vi "Set Value.vi"(0 "Diagram in":refnum<vi>, 1 "Sub Items":T1[](array[typedef]), 5 "Value in":refnum<vi>, 9 "Input Terms in":cluster{refnum<vi>, "Type":variant}[](array[cluster]), 11 "error in (no error)":errorcluster) -> (4 "Diagram out":refnum<vi>, 6 "Value out":refnum<vi>, 8 "Equal":refnum<vi>, 10 "Input Terms out":cluster{refnum<vi>, "Type":variant}[](array[cluster]), 15 "error out":errorcluster)   [LabVIEW 2015, in "Read-Write-Signals.xnode"]
uses:
  Read-Write-Signals.xnode
  Read-Write-Signals Sub Item.ctl
  Read-Write-Signals Sub Item Type.ctl
  <vilib>/Erdos Miller/LV-Scripting/LV-Scripting.lvlib
  <vilib>/Utility/Data Type/NI_Data Type.lvlib
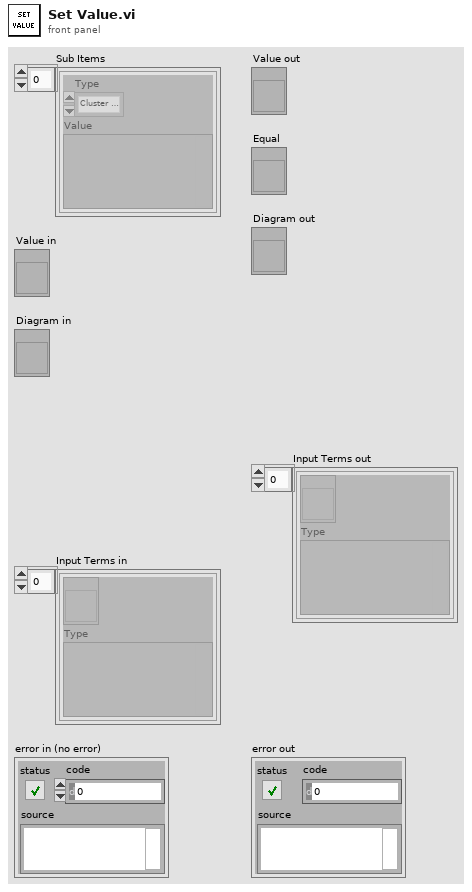
[diagram p1: front panel]
types:
  T1 = typedef "Read-Write-Signals Sub Item.ctl" = cluster{"Type":T2, "Value":variant}
  T2 = typedef "Read-Write-Signals Sub Item Type.ctl" = enum8{"Cluster Element", "Array Element", "Subarray"}
  T3 = cluster{"Outer Term":refnum<vi>, "Type":variant}[]
  T4 = typedef "NI_Data Type.lvlib/Data Type.ctl" = enum8{"Invalid Type", "Void", "I8", "I16", "I32", "I64", "U8", "U16", "U32", "U64", "Single Float", "Double Float", "Extended Float", "Single Complex", "Double Complex", "Extended Complex", "Enum U8", "Enum U16", "Enum U32", "Enum U64", "Single Float With Unit", "Double Float With Unit", "Extended Float With Unit", "Single Complex with Unit", "Double Complex with Unit", "Extended Complex with Unit", "Boolean", "String", "Path", "Picture", "Tag", "Array", "Cluster", "Variant", "LV Variant", "Waveform", "Timestamp", "Digital Waveform", "Digital Data", "ExpressData", "Refnum", "External Data", "VI", "Poly VI", "LabVIEW Class Instance", "Fixed Point"}
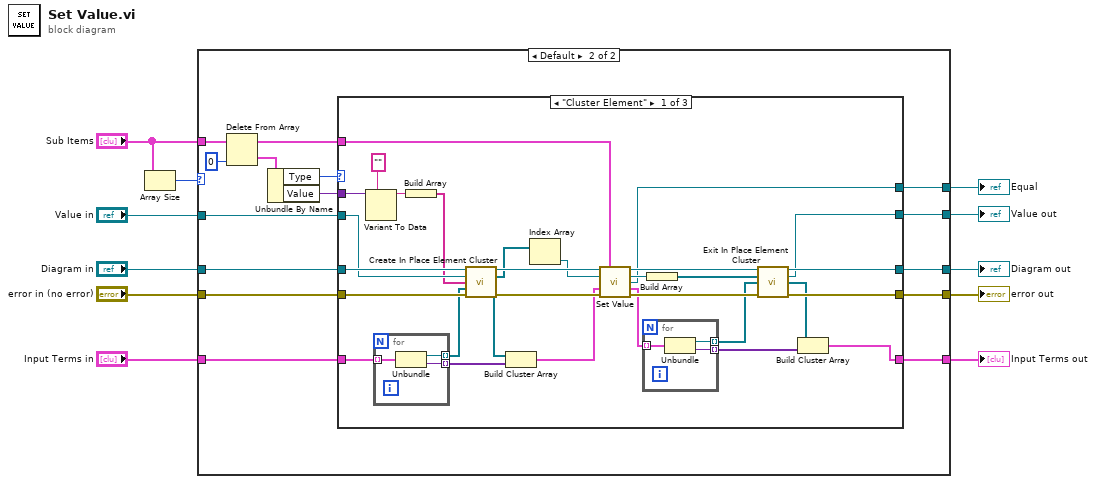
[diagram p0: block diagram]
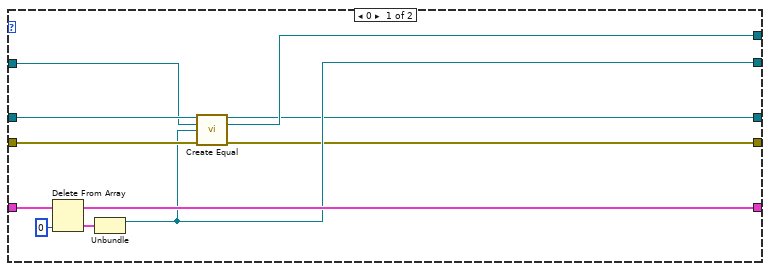
[diagram p2: hidden frame]
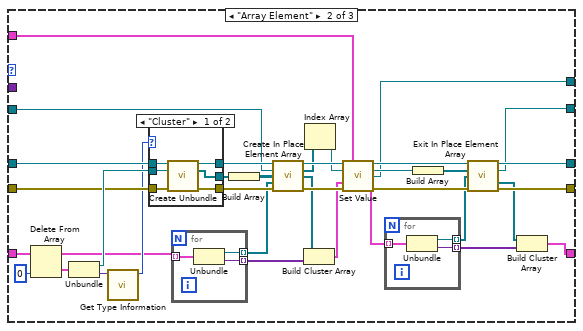
[diagram p3: hidden frame]
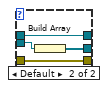
[diagram p4: hidden frame]
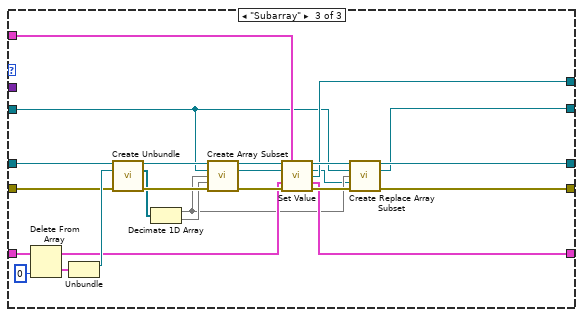
[diagram p5: hidden frame]
diagram:
  n1 = Array Size(array="Sub Items") -> (size(s)=w2:i32)
  n2 = case shown="Default" w2 {
    tunnel: [w14 w37] -> w11
    tunnel: "Sub Items" -> [_ w26]
    tunnel: [w15 w34] -> w10
    tunnel: [w12 w33] -> w9
    tunnel: "error in (no error)" -> [w22 w32]
    tunnel: "Diagram in" -> [w21 w31]
    tunnel: [w18 w30] -> w6
    tunnel: [w13 w29] -> w5
    tunnel: "Input Terms in" -> [w20 w28]
    tunnel: "Value in" -> [w16 w27]
    frame 0 {
      n3 = Delete From Array(array=w20, index=0) -> (deleted portion=w17:cluster{refnum<vi>, "Type":variant}, array with subset deleted=w18:cluster{refnum<vi>, "Type":variant}[])  [unwired: 1 in]
      n4 = Unbundle(w17) -> (w15:refnum<vi>)  [unwired: 1 out]
      n5 = call <vilib>:"Create Equal.vi"("Diagram in"=w21, "x"=w16, "y"=w15, "error in (no error)"=w22) -> ("Diagram out"=w12:refnum<vi>, "x = y?"=w14:refnum<vi>, "error out"=w13:errorcluster)  [unwired: 9 in]
    }
    frame Default {
      n6 = Delete From Array(array=w26, index=0) -> (deleted portion=w23:T1, array with subset deleted=w24:T1[])  [unwired: 1 in]
      n7 = Unbundle By Name(w23) -> ("Type"=w35:T2, "Value"=w36:variant)
      n8 = case shown="\"Cluster Element\"" w35 {
        tunnel: w36 -> [w67 _ _]
        tunnel: w28 -> [w47 w109 w150]
        tunnel: w31 -> [w64 w106 w147]
        tunnel: w32 -> [w63 w105 w146]
        tunnel: [w38 w74 w132] -> w30
        tunnel: [w52 w87 w140] -> w33
        tunnel: [w54 w85 w141] -> w29
        tunnel: w27 -> [w62 w98 w128]
        tunnel: [w48 w86 w129] -> w34
        tunnel: [w49 w84 w130] -> w37
        tunnel: w24 -> [w56 w95 w135]
        frame "Cluster Element" {
          n9 = Variant To Data(type="", Variant=w67) -> (data=w65:string)  [unwired: 1 in, 1 out]
          n10 = for {
            tunnel: w47 -> [w73] mode=indexing
            tunnel: [w72] -> w46 mode=indexing
            tunnel: [w71] -> w45 mode=indexing
            n11 = Unbundle(w73) -> (w72:refnum<vi>, "Type"=w71:variant)
          }
          n12 = Build Array(w65) -> (w61:string[])
          n13 = call <vilib>:"Create In Place Element Cluster.vi"("Diagram in"=w64, "Cluster"=w62, "Element Names"=w61, "Inputs"=w46, "error in (no error)"=w63) -> ("Diagram out"=w60:refnum<vi>, "Elements"=w59:refnum<vi>[], "Inputs"=w44:refnum<vi>[], "error out"=w57:errorcluster)  [unwired: 7 in]
          n14 = Build Cluster Array(w44, w45) -> (w43:cluster{refnum<vi>, "Type":variant}[])
          n15 = Index Array(array=w59) -> (element=w58:refnum<vi>)  [unwired: 1 in]
          n16 = call "Set Value.vi"("Diagram in"=w60, "Sub Items"=w56, "Value in"=w58, "Input Terms in"=w43, "error in (no error)"=w57) -> ("Diagram out"=w53:refnum<vi>, "Value out"=w51:refnum<vi>, "Equal"=w49:refnum<vi>, "Input Terms out"=w41:cluster{refnum<vi>, "Type":variant}[], "error out"=w55:errorcluster)  [unwired: 6 in]
          n17 = for {
            tunnel: w41 -> [w70] mode=indexing
            tunnel: [w69] -> w40 mode=indexing
            tunnel: [w68] -> w42 mode=indexing
            n18 = Unbundle(w70) -> (w69:refnum<vi>, "Type"=w68:variant)
          }
          n19 = Build Array(w51) -> (w50:refnum<vi>[])
          n20 = call <vilib>:"Exit In Place Element Cluster.vi"("Diagram in"=w53, "Elements"=w50, "Outputs"=w40, "error in (no error)"=w55) -> ("Diagram out"=w52:refnum<vi>, "Cluster"=w48:refnum<vi>, "Outputs"=w39:refnum<vi>[], "error out"=w54:errorcluster)  [unwired: 8 in]
          n21 = Build Cluster Array(w39, w42) -> (w38:T3)
        }
        frame "Array Element" {
          n22 = Delete From Array(array=w109, index=0) -> (deleted portion=w108:cluster{refnum<vi>, "Type":variant}, array with subset deleted=w82:cluster{refnum<vi>, "Type":variant}[])  [unwired: 1 in]
          n23 = Unbundle(w108) -> (w107:refnum<vi>, "Type"=w103:variant)
          n24 = call <vilib>:"Get Type Information.vi"("Variant"=w103) -> ("Type"=w102:T4)  [unwired: 6 in, 4 out]
          n25 = case shown="\"Cluster\"" w102 {
            tunnel: w107 -> [w119 w125]
            tunnel: w106 -> [w121 w123]
            tunnel: w105 -> [w120 w124]
            tunnel: [w117 w124] -> w100
            tunnel: [w118 w123] -> w99
            tunnel: [w116 w122] -> w104
            frame "Cluster" {
              n26 = call <vilib>:"Create Unbundle.vi"("Diagram in"=w121, "input cluster"=w119, "error in (no error)"=w120) -> ("Diagram out"=w118:refnum<vi>, "Outputs"=w116:refnum<vi>[], "error out"=w117:errorcluster)  [unwired: 10 in]
            }
            frame Default {
              n27 = Build Array(w125) -> (w122:refnum<vi>[])
            }
          }
          n28 = for {
            tunnel: w82 -> [w115] mode=indexing
            tunnel: [w114] -> w81 mode=indexing
            tunnel: [w113] -> w83 mode=indexing
            n29 = Unbundle(w115) -> (w114:refnum<vi>, "Type"=w113:variant)
          }
          n30 = Build Array(w104) -> (w97:refnum<vi>[][])
          n31 = call <vilib>:"Create In Place Element Array.vi"("Diagram in"=w99, "Array"=w98, "Indices"=w97, "Inputs"=w81, "error in (no error)"=w100) -> ("Diagram out"=w96:refnum<vi>, "Elements"=w93:refnum<vi>[], "Inputs"=w80:refnum<vi>[], "error out"=w94:errorcluster)  [unwired: 7 in]
          n32 = Build Cluster Array(w80, w83) -> (w79:cluster{refnum<vi>, "Type":variant}[])
          n33 = Index Array(array=w93) -> (element=w92:refnum<vi>)  [unwired: 1 in]
          n34 = call "Set Value.vi"("Diagram in"=w96, "Sub Items"=w95, "Value in"=w92, "Input Terms in"=w79, "error in (no error)"=w94) -> ("Diagram out"=w90:refnum<vi>, "Value out"=w91:refnum<vi>, "Equal"=w84:refnum<vi>, "Input Terms out"=w77:cluster{refnum<vi>, "Type":variant}[], "error out"=w88:errorcluster)  [unwired: 6 in]
          n35 = for {
            tunnel: w77 -> [w112] mode=indexing
            tunnel: [w111] -> w76 mode=indexing
            tunnel: [w110] -> w78 mode=indexing
            n36 = Unbundle(w112) -> (w111:refnum<vi>, "Type"=w110:variant)
          }
          n37 = Build Array(w91) -> (w89:refnum<vi>[])
          n38 = call <vilib>:"Exit In Place Element Array.vi"("Diagram in"=w90, "Elements"=w89, "Outputs"=w76, "error in (no error)"=w88) -> ("Diagram out"=w87:refnum<vi>, "Array"=w86:refnum<vi>, "Outputs"=w75:refnum<vi>[], "error out"=w85:errorcluster)  [unwired: 7 in, 1 out]
          n39 = Build Cluster Array(w75, w78) -> (w74:T3)
        }
        frame "Subarray" {
          n40 = Delete From Array(array=w150, index=0) -> (deleted portion=w149:cluster{refnum<vi>, "Type":variant}, array with subset deleted=w133:cluster{refnum<vi>, "Type":variant}[])  [unwired: 1 in]
          n41 = Unbundle(w149) -> (w148:refnum<vi>)  [unwired: 1 out]
          n42 = call <vilib>:"Create Unbundle.vi"("Diagram in"=w147, "input cluster"=w148, "error in (no error)"=w146) -> ("Diagram out"=w144:refnum<vi>, "Outputs"=w142:refnum<vi>[], "error out"=w145:errorcluster)  [unwired: 10 in]
          n43 = Decimate 1D Array(w142) -> (w131:refnum<vi>[], w143:refnum<vi>[])
          n44 = call <vilib>:"Create Array Subset.vi"("Diagram in"=w144, "array"=w128, "Indices"=w131, "Lengths"=w143, "error in (no error)"=w145) -> ("Diagram out"=w139:refnum<vi>, "subarray"=w134:refnum<vi>, "error out"=w137:errorcluster)  [unwired: 8 in]
          n45 = call "Set Value.vi"("Diagram in"=w139, "Sub Items"=w135, "Value in"=w134, "Input Terms in"=w133, "error in (no error)"=w137) -> ("Diagram out"=w138:refnum<vi>, "Value out"=w127:refnum<vi>, "Equal"=w130:refnum<vi>, "Input Terms out"=w132:cluster{refnum<vi>, "Type":variant}[], "error out"=w136:errorcluster)  [unwired: 6 in]
          n46 = call <vilib>:"Create Replace Array Subset.vi"("Diagram in"=w138, "array"=w128, "Indices"=w131, "new element/subarray"=w127, "error in (no error)"=w136) -> ("Diagram out"=w140:refnum<vi>, "output array"=w129:refnum<vi>, "error out"=w141:errorcluster)  [unwired: 8 in]
        }
      }
    }
  }
  "Equal" <- w11
  "Value out" <- w10
  "Diagram out" <- w9
  "Input Terms out" <- w6
  "error out" <- w5
